vi "脉冲生成_基于频率_有限.vi"() -> ()   [LabVIEW 2013]
uses:
  <userlib>/ArtDAQ/_SubVI/ArtDAQ_CreateCOPulseChanFreq.vi
  <userlib>/ArtDAQ/_SubVI/ArtDAQ_CfgImplicitTiming.vi
  <userlib>/ArtDAQ/_SubVI/ArtDAQ_CfgDigEdgeStartTrig.vi
panel:
  in  "触发模式":enum32{"No Trigger", "DigStartTrig"}(tab)=enum."DigStartTrig"
  in  "可重?":bool
  in  "触发边沿":i32(ring)=10280 items=["上升"=10280, "下降"=10171]
  in  "触发源":string(combo)="/Dev1/PFI1"
  in  "每通道采样数":i32=100
  in  "Stop":bool
  in  "计数器":string="Dev1/ctr0"
  in  "占空比":dbl=0.5 format="%0.6f"
  in  "频率":dbl=100.0 format="%0.6f"
  out "错误输出":errorcluster
  # "通道属性"
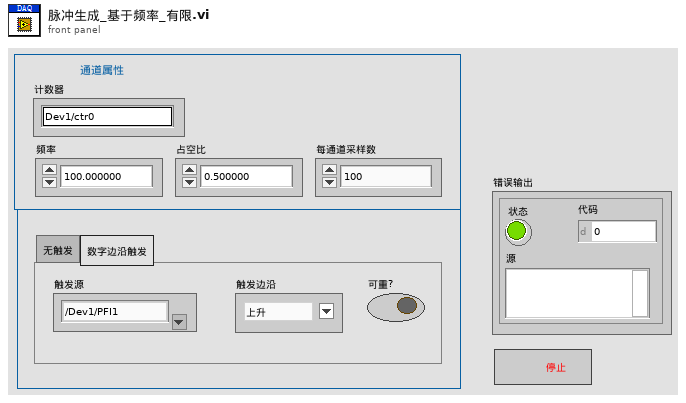
[diagram p1: front panel]
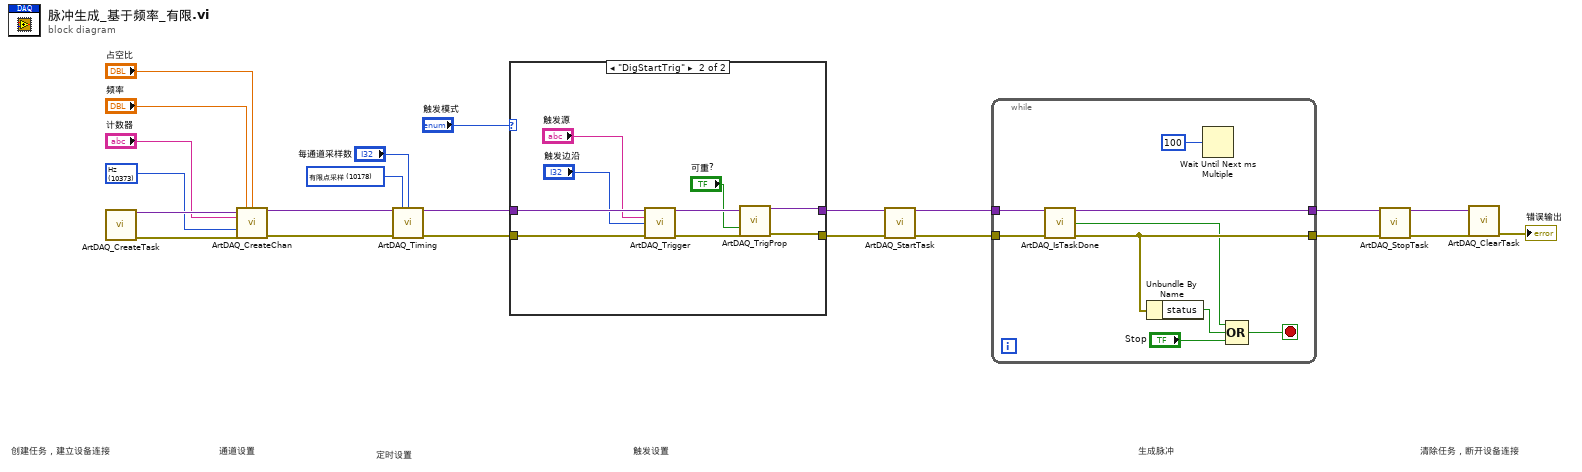
[diagram p0: block diagram]
diagram:
  w8 = 10373 items=["Hz"=10373] ("Units")
  w10 = 10178 items=["有限点采样"=10178, "连续采样"=10123] ("SampleMode")
  # "定时设置"
  # "清除任务，断开设备连接"
  # "生成脉冲"
  # "触发设置"
  # "通道设置"
  # "创建任务，建立设备连接"
  n1 = call <userlib>:"ArtDAQ_CreateTask.vi"() -> ("任务句柄"=w22:variant, "错误输出"=w21:errorcluster)  [unwired: 14 in]
  n2 = call-poly <userlib>:"ArtDAQ_CreateChan.vi"("任务句柄"=w22, "频率"="频率", "占空比"="占空比", "计数器"="计数器", "单位"=w8, "错误输入"=w21) -> ("任务句柄"=w12:variant, "错误输出"=w11:errorcluster)  [unwired: 8 in]
  n3 = call-poly <userlib>:"ArtDAQ_Timing.vi"("任务句柄"=w12, "采样模式"=w10, "每通道采样数"="每通道采样数", "错误输入"=w11) -> ("任务句柄"=w1:variant, "错误输出"=w2:errorcluster)  [unwired: 10 in]
  n4 = case shown="\"DigStartTrig\"" "触发模式" {
    tunnel: w1 -> [w24 w33]
    tunnel: [w24 w26] -> w6
    tunnel: [w23 w28] -> w4
    tunnel: w2 -> [w23 w32]
    frame "No Trigger", Default {
    }
    frame "DigStartTrig" {
      n5 = call-poly <userlib>:"ArtDAQ_Trigger.vi"("任务句柄"=w33, "触发源"="触发源", "边沿"="触发边沿", "错误输入"=w32) -> ("任务句柄"=w27:variant, "错误输出"=w29:errorcluster)  [unwired: 10 in]
      n6 = call-poly <userlib>:"ArtDAQ_TrigProp.vi"("任务句柄"=w27, "可重?"="可重?", "错误输入"=w29) -> ("任务句柄"=w26:variant, "错误输出"=w28:errorcluster)  [unwired: 11 in]
    }
  }
  n7 = call <userlib>:"ArtDAQ_StartTask.vi"("任务句柄"=w6, "错误输入"=w4) -> ("任务句柄"=w5:variant, "错误输出"=w3:errorcluster)  [unwired: 12 in]
  n8 = while {
    tunnel: [w42] -> w19
    tunnel: [w41] -> w17
    tunnel: w5 -> [w38]
    tunnel: w3 -> [w37]
    stop <- w36 stop-if-true
    n9 = call <userlib>:"ArtDAQ_IsTaskDone.vi"("任务句柄"=w38, "错误输入"=w37) -> ("任务句柄"=w42:variant, "完成任务？"=w34:bool, "错误输出"=w41:errorcluster)  [unwired: 11 in]
    n10 = Unbundle By Name(w41) -> ("status"=w40:bool)
    n11 = Wait Until Next ms Multiple(millisecond multiple=u32 100 ("毫秒倍数")) -> ()  [unwired: 1 out]
    n12 = Compound Arithmetic op=OR(w34, w40, "Stop") -> (w36:bool)
  }
  n13 = call <userlib>:"ArtDAQ_StopTask.vi"("任务句柄"=w19, "错误输入"=w17) -> ("任务句柄"=w18:variant, "错误输出"=w16:errorcluster)  [unwired: 12 in]
  n14 = call <userlib>:"ArtDAQ_ClearTask.vi"("任务句柄"=w18, "错误输入"=w16) -> ("错误输出"=→"错误输出":errorcluster)  [unwired: 13 in]
